vi "Analyze Quantized Filter with Different Structure.vi"() -> ()   [LabVIEW 2023]
doc: "Demonstrates the effects of different filter structures on coefficients quantization.\n\nComplete the following steps to use this VI.\n1) Run the VI.\n2) Leave the Coefficients Quantization Settings unchanged. Select a different <B>Target Structure</B>.\n3) Observe the Magnitude Responses and Coefficients Report outputs to see the effect.\n4) Select <B>IIR Direct Form II</B> from <B>Target Structure</B>, and modify the integer word length (<B>iwl</B>).\n5) Observe the Magnitude Responses and Coefficients Report outputs to see the effect.\n6) Click the <B>STOP</B> button to stop this VI."
uses:
  <vilib>/addons/Digital Filter Design/_Objects.llb/DFD Quantization Settings.ctl
  <vilib>/addons/Digital Filter Design/_Objects.llb/DFD Quantization Sources.ctl
  <vilib>/addons/Digital Filter Design/_Objects.llb/DFD Filter Frequence Specification (Design).ctl
  <vilib>/addons/Digital Filter Design/_Objects.llb/DFD Filter Ripple Specification (Design).ctl
  <vilib>/addons/Digital Filter Design/FXPModel.llb/DFD FXP Quantize Coef (Advanced).vi
  <vilib>/addons/Digital Filter Design/Analysis.llb/DFD Plot Freq Response (Linear-Spaced).vi
  <vilib>/addons/Digital Filter Design/NI_DigFilterLicensed.lvlib
panel:
  in  "Target Structure":u16(ring)=21 items=["FIR Direct Form"=1, "FIR Direct Form Transposed"=2, "FIR Symmetric"=3, "FIR Antisymmetric"=4, "IIR Direct Form I"=5, "IIR Direct Form I Transposed"=6, "IIR Direct Form II"=7, "IIR Direct Form II Transposed"=8, "IIR Cascaded Second-Order Sections Form I"=9, "IIR Cascaded Second-Order Sections Form I Transposed"=10, "IIR Cascaded Second-Order Sections Form II"=11, "IIR Cascaded Second-Order Sections Form II Transposed"=12, "Lattice Allpass (basic sections)"=13, "Lattice Allpass (one multiplier sections)"=14, "Lattice Allpass (normalized sections)"=15, "Lattice AR (basic sections)"=16, "Lattice AR (one multiplier sections)"=17, "Lattice AR (normalized sections)"=18, "Lattice MA (minimum phase)"=19, "Lattice MA (maximum phase)"=20, "Lattice ARMA (basic sections)"=21, "Lattice ARMA (one multiplier sections)"=22, "Lattice ARMA (normalized sections)"=23]
  in  "Coefficients Quantizer":T1={"source"=0, "wl"=16, "iwl"=1, "overflow mode"=enum."Saturation", "rounding mode"=enum."Nearest", "signed?"=TRUE} {"source" items=["Coefficients a/k"=0, "Coefficients b/v"=7, "Input"=1, "Output"=2, "Multiplicand"=3, "Product"=4, "Sum"=5, "Delay"=6]}
  out "Error Message":string
  in  "Instructions":string="1. Leave the coefficients quantization settings unchanged. Select a different structure to see the effect.\n\n2. Select the IIR Direct II structure, modify the integer word length (iwl) to see the effect."
  in  "stop":bool
  out "Coefficients Report":string
  out "Magnitude Responses":cluster{"f0":dbl, "df":dbl, "values":dbl[]}[](graph)
  # "Select Help>>Show Context Help and move the cursor over the VI icon for more information."
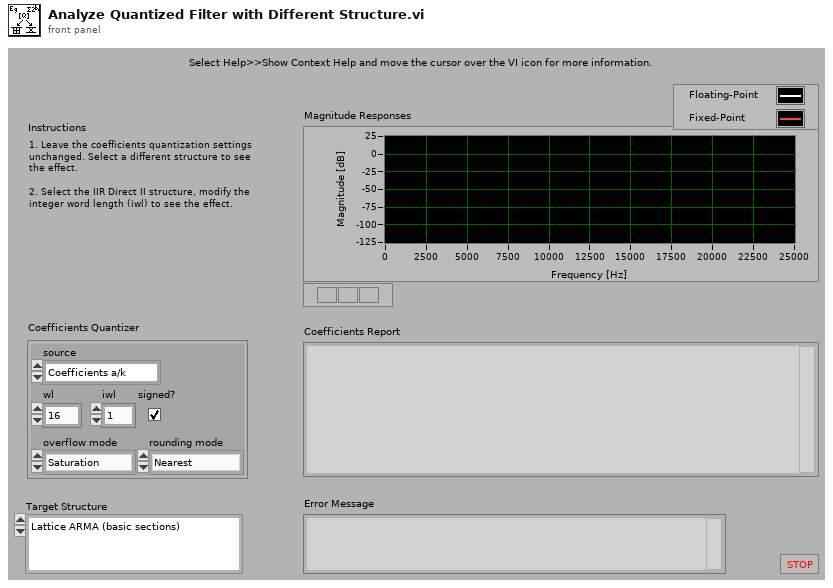
[diagram p1: front panel]
types:
  T1 = typedef "NI_DigFilterLicensed.lvlib/DFD Quantization Settings.ctl" = cluster{"source":T2, "wl":i16, "iwl":i16, "overflow mode":enum16{"Saturation", "Wrap"}, "rounding mode":enum16{"Nearest", "Truncation"}, "signed?":bool}
  T2 = typedef "NI_DigFilterLicensed.lvlib/DFD Quantization Sources.ctl" = u16
  T3 = typedef "NI_DigFilterLicensed.lvlib/DFD Filter Ripple Specification (Design).ctl" = cluster{"passband":dbl, "stopband":dbl, "dB/linear? (T: dB)":bool}
  T4 = typedef "NI_DigFilterLicensed.lvlib/DFD Filter Frequence Specification (Design).ctl" = cluster{"fpass 1":dbl, "fstop 1":dbl, "fpass 2 ":dbl, "fstop 2":dbl}
  T5 = typedef "NI_DigFilterLicensed.lvlib/DFD Filter Obj.ctl" = cluster{"mSRate_Fs":dbl, "mSRate_Version":string, "mSRate_Comments":string, "mSRate_OrgCoef":T6, "mSRate_CurCoef":T6, "mSRate_Quantized?":bool, "mSRate_QCoef":T6, "mSRate_QSettings":T8[], "mSRate_Order":i32, "mSRate_Scaling":cluster{"mSRate_ScaleByPowerOf2?":bool, "mSRate_ScaleType":T10}}
  T6 = typedef "NI_DigFilterLicensed.lvlib/DFD Filter Coef.ctl" = cluster{"type":T7, "gain":dbl, "coef a (k)":dbl[], "coef b (v)":dbl[]}
  T7 = typedef "NI_DigFilterLicensed.lvlib/DFD Filter Structure Type Selector.ctl" = enum16{"Undefined", "FIR Direct Form", "FIR Direct Form Transposed", "FIR Symmetric", "FIR Antisymmetric", "IIR Direct Form I", "IIR Direct Form I Transposed", "IIR Direct Form II", "IIR Direct Form II Transposed", "IIR Cascaded Second Order Sections Form I", "IIR Cascaded Second Order Sections Form I Transposed", "IIR Cascaded Second Order Sections Form II", "IIR Cascaded Second Order Sections Form II Transposed", "Lattice Allpass (basic sections)", "Lattice Allpass (one multiplier sections)", "Lattice Allpass (normalized sections)", "Lattice AR (basic sections)", "Lattice AR (one multiplier sections)", "Lattice AR (normalized sections)", "Lattice MA (minimum phase)", "Lattice MA (maximum phase)", "Lattice ARMA (basic sections)", "Lattice ARMA (one multiplier sections)", "Lattice ARMA (normalized sections)"}
  T8 = typedef "NI_DigFilterLicensed.lvlib/dfd_Internal Quantization Settings.ctl" = cluster{"source":T9, "wl":i16, "iwl":i16, "overflow mode":enum16{"Saturation", "Wrap"}, "rounding mode":enum16{"Nearest", "Truncation"}, "signed?":bool}
  T9 = typedef "NI_DigFilterLicensed.lvlib/dfd_Internal Quantization Srcs.ctl" = u16
  T10 = typedef "NI_DigFilterLicensed.lvlib/DFD Coef Norm Type.ctl" = enum16{"No Norm", "Time Domain 1-Norm", "Time Domain 2-Norm", "Time Domain Inf-Norm"}
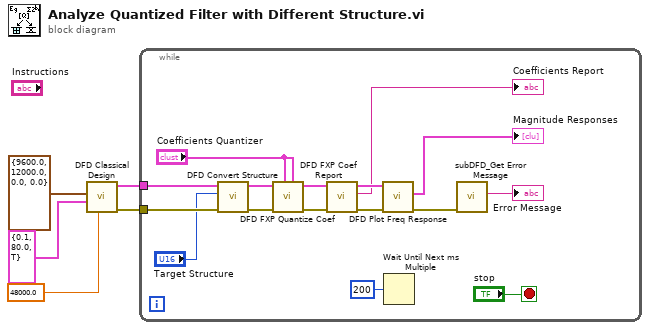
[diagram p0: block diagram]
diagram:
  n1 = call <vilib>:"DFD Classical Design.vi"("fs [Hz]"=48000.0, "ripple specs"=T3 {"passband"=0.1, "stopband"=80.0, "dB/linear? (T: dB)"=TRUE}, "freq specs [Hz]"=T4 {"fpass 1"=9600.0, "fstop 1"=12000.0, "fpass 2 "=0.0, "fstop 2"=0.0}) -> ("error out"=w4:errorcluster, "filter out"=w5:T5)  [unwired: 3 in, 4 out]
  n2 = while {
    tunnel: w5 -> [w13]
    tunnel: w4 -> [w12]
    stop <- "stop" stop-if-true
    n3 = call <vilib>:"DFD Convert Structure.vi"("error in (no error)"=w12, "target structure"="Target Structure", "filter in"=w13) -> ("error out"=w20:errorcluster, "filter out"=w21:T5)  [unwired: 7 out]
    n4 = call-poly <vilib>:"DFD FXP Quantize Coef.vi"("coefficients b/v quantizer"="Coefficients Quantizer", "coefficients a/k quantizer"="Coefficients Quantizer", "error in (no error)"=w20, "filter in"=w21) -> ("error out"=w18:errorcluster, "filter out"=w19:T5)  [unwired: 1 in, 5 out]
    n5 = call <vilib>:"DFD FXP Coef Report.vi"("error in (no error)"=w18, "filter in"=w19) -> ("error out"=w16:errorcluster, "coefficients report"=→"Coefficients Report":string, "filter out"=w17:T5)  [unwired: 7 out]
    n6 = call-poly <vilib>:"DFD Plot Freq Response.vi"("error in (no error)"=w16, "filter in"=w17) -> ("error out"=w8:errorcluster, "magnitude response"=→"Magnitude Responses":cluster{"f0":dbl, "df":dbl, "values":dbl[]}[])  [unwired: 6 in, 2 out]
    n7 = Wait Until Next ms Multiple(millisecond multiple=u32 200) -> ()  [unwired: 1 out]
    n8 = call <vilib>:"subDFD_Get Error Message.vi"("error in (no error)"=w8) -> ("Error Message"=→"Error Message":string)  [unwired: 10 out]
  }
